vi "ParseText.vi"(11 "text":string) -> (1 "int":i32, 3 "Posit Array":T1[](array[typedef]))   [LabVIEW 2014]
uses:
  Libraries/Contact Data/Position.ctl
  Libraries/Contact Data/Contact Data.lvlib
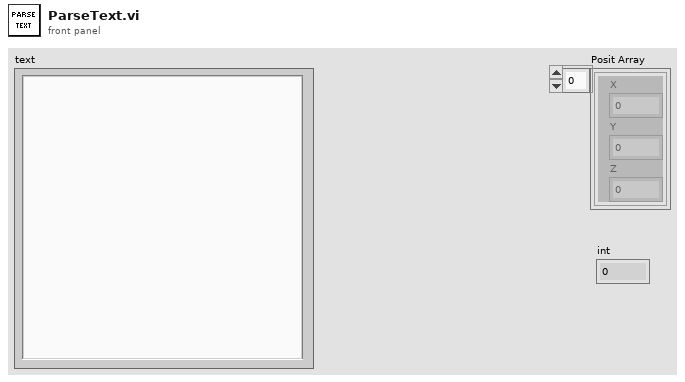
[diagram p1: front panel]
types:
  T1 = typedef "Contact Data.lvlib/Position.ctl" = cluster{"X":dbl, "Y":dbl, "Z":dbl}
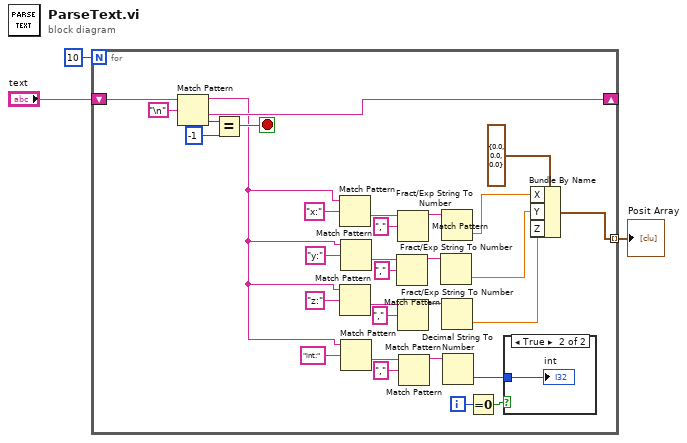
[diagram p0: block diagram]
diagram:
  n1 = for {
    N: 10 -> [_]
    shift-right: [w13] -> _
    shift-left: "text" -> [w33]
    tunnel: [w7] -> w1 mode=indexing
    i -> [w5]
    stop <- w30 stop-if-true
    n2 = Match Pattern(string=w33, regular expression="\n") -> (before substring=w12:string, after substring=w13:string, offset past match=w32:i32)  [unwired: 1 in, 1 out]
    n3 = Equal?(x=w32, y=-1) -> (x = y?=w30:bool)
    n4 = Match Pattern(string=w12, regular expression="x:" ("format string")) -> (after substring=w16:string)  [unwired: 1 in, 3 out]
    n5 = Match Pattern(string=w12, regular expression="z:" ("format string")) -> (after substring=w24:string)  [unwired: 1 in, 3 out]
    n6 = Match Pattern(string=w12, regular expression="y:" ("format string")) -> (after substring=w19:string)  [unwired: 1 in, 3 out]
    n7 = Match Pattern(string=w12, regular expression="int:" ("format string")) -> (after substring=w27:string)  [unwired: 1 in, 3 out]
    n8 = Match Pattern(string=w19, regular expression=",") -> (before substring=w21:string)  [unwired: 1 in, 3 out]
    n9 = Match Pattern(string=w16, regular expression=",") -> (before substring=w14:string)  [unwired: 1 in, 3 out]
    n10 = Match Pattern(string=w24, regular expression=",") -> (before substring=w22:string)  [unwired: 1 in, 3 out]
    n11 = Match Pattern(string=w27, regular expression=",") -> (before substring=w29:string)  [unwired: 1 in, 3 out]
    n12 = Fract/Exp String To Number(string=w21) -> (number=w9:dbl)  [unwired: 3 in, 1 out]
    n13 = Fract/Exp String To Number(string=w14) -> (number=w10:dbl)  [unwired: 3 in, 1 out]
    n14 = Fract/Exp String To Number(string=w22) -> (number=w8:dbl)  [unwired: 3 in, 1 out]
    n15 = Decimal String To Number(string=w29) -> (number=w6:i32)  [unwired: 2 in, 1 out]
    n16 = Equal To 0?(x=w5) -> (x = 0?=w4:bool)
    n17 = case shown="True" w4 {
      tunnel: w6 -> [_ w35]
      frame False {
      }
      frame True {
        "int" <- w35
      }
    }
    n18 = Bundle By Name(cluster=T1 {"X"=0.0, "Y"=0.0, "Z"=0.0} ("Position"), "X"=w10, "Y"=w9, "Z"=w8) -> (w7:T1)
  }
  "Posit Array" <- w1
